vi "Updated Command Status.vi"(8 "error in (no error)":errorcluster, 10 "Command Status":T1, 11 "Command Processor in":refnum<class "Command Processor Actor.lvclass">) -> (0 "error out":errorcluster, 3 "Command Processor out":refnum<class "Command Processor Actor.lvclass">)   [LabVIEW 2014, in "Robot Actor Framework.lvlib" / "Command Processor Actor.lvlib" / "Command Processor Actor.lvclass"]
uses:
  Command Processor Actor.lvclass
  Command Actor/Command Actor Class/Command State.ctl
  Command Actor/Command Actor Class/Command States.ctl
  <vilib>/ActorFramework/Actor/Actor.lvclass/Actor.ctl
  System Actor/System Actor Messages/Updated Command Status Msg/Updated Command Status Msg.lvclass/Updated Command Status Msg.ctl
  <vilib>/ActorFramework/Message Enqueuer/Message Enqueuer.lvclass/Message Enqueuer.ctl
  <vilib>/ActorFramework/Message Enqueuer/Enqueue.vi
  <vilib>/ActorFramework/Message Priority Queue/Priority Enqueue.vi
  System Actor/System Actor Messages/Updated Command Status Msg/Updated Command Status Msg.lvclass
  <vilib>/ActorFramework/Actor/Actor.lvclass
  Command Actor/Command Actor Class/Command Actor.lvclass
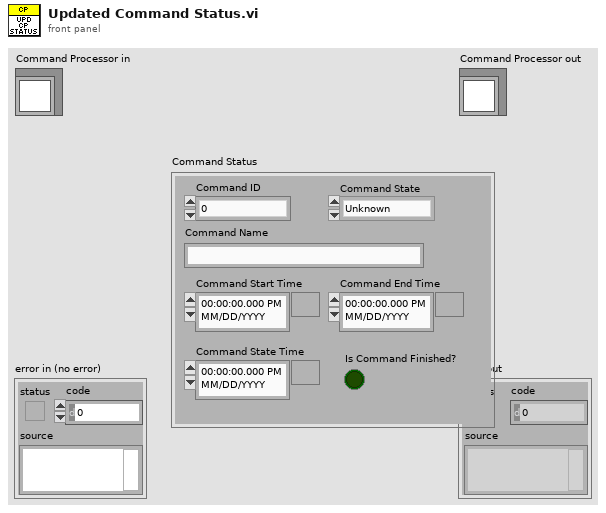
[diagram p1: front panel]
types:
  T1 = typedef "Robot Actor Framework.lvlib/Command Actor.lvlib/Command Actor.lvclass/Command State.ctl" = cluster{"Command Name":string, "Command Start Time":timestamp, "Command End Time":timestamp, "Is Command Finished?":bool, "Command ID":u32, "Command State":T2, "Command State Time":timestamp}
  T2 = typedef "Robot Actor Framework.lvlib/Command Actor.lvlib/Command Actor.lvclass/Command States.ctl" = enum16{"Unknown", "Started", "Stopped", "Finished"}
  T3 = typedef "Robot Actor Framework.lvlib/Command Processor Actor.lvlib/Command Processor Actor.lvclass/Command Processor State.ctl" = cluster{"Current State":T4, "Last State Update":timestamp, "Queued Commands":u32, "Current Command Status":T1, "Previous State":T4, "Current State Entry":timestamp, "Transitioning State":bool, "Commands Behind":dbl, "Last Command Queue Time":timestamp}
  T4 = typedef "Robot Actor Framework.lvlib/Command Processor Actor.lvlib/Command Processor Actor.lvclass/Command Processor States.ctl" = enum16{"Unknown", "No Command", "Running Command", "Starting Command", "Stopping Command", "Finishing Command"}
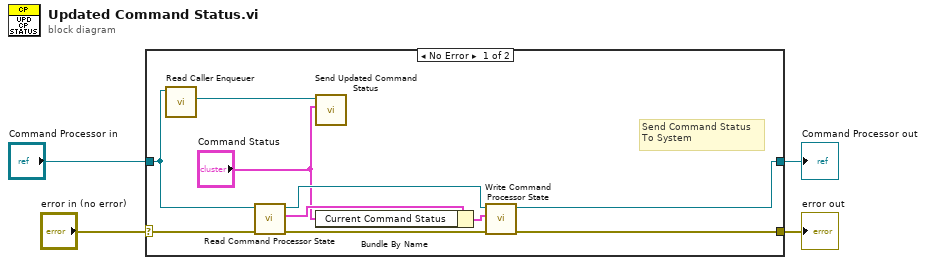
[diagram p0: block diagram]
diagram:
  n1 = case shown="No Error" "error in (no error)" {
    selector: "error in (no error)" -> [w7 w16]
    tunnel: [w5 w16] -> w3
    tunnel: [w14 w15] -> w1
    tunnel: "Command Processor in" -> [w10 w15]
    frame No Error {
      # "Send Command Status\nTo System"
      n2 = call <vilib>:"Read Caller Enqueuer.vi"("Actor"=w10) -> ("Caller Enqueuer"=w9:refnum<class "Message Enqueuer.lvclass">)  [unwired: 10 in]
      n3 = call-dynamic "Read Command Processor State.vi"("error in (no error)"=w7, "Command Processor in"=w10) -> ("error out"=w6:errorcluster, "Command Processor State"=w12:T3, "Command Processor out"=w13:refnum<class "Command Processor Actor.lvclass">)  [unwired: 7 in]
      n4 = call "Send Updated Command Status.vi"("Command Status"="Command Status", "Message Enqueuer"=w9) -> ()  [unwired: 8 in, 2 out]
      n5 = Bundle By Name(cluster=w12, "Current Command Status"="Command Status") -> (w11:T3)
      n6 = call-dynamic "Write Command Processor State.vi"("error in (no error)"=w6, "Command Processor State"=w11, "Command Processor in"=w13) -> ("error out"=w5:errorcluster, "Command Processor out"=w14:refnum<class "Command Processor Actor.lvclass">)  [unwired: 7 in]
    }
    frame Error {
    }
  }
  "error out" <- w3
  "Command Processor out" <- w1
